vi "M--front RSw.vi"(8 "Command Info In":T1, 10 "M--front RSw":T4) -> (0 "Command Info Out":T1)   [LabVIEW 2017]
uses:
  Block Clusters/M--front RSw.ctl
  <vilib>/Rock Robotics/WPI/Framework/Command Status Info.ctl
  <vilib>/Rock Robotics/WPI/Framework/Completion Status.ctl
  <vilib>/Rock Robotics/WPI/Framework/Completion Notifier.ctl
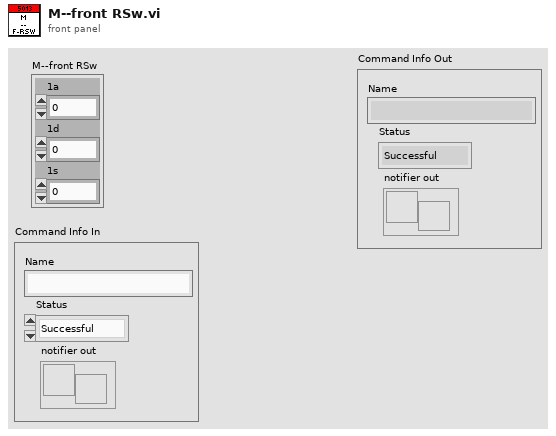
[diagram p1: front panel]
types:
  T1 = typedef "Command Status Info.ctl" = cluster{"Name":string, "Status":T2, "notifier out":T3}
  T2 = typedef "Completion Status.ctl" = enum16{"Successful", "Aborted", "Incomplete"}
  T3 = typedef "Completion Notifier.ctl" = refnum<notifier>
  T4 = typedef "M--front RSw.ctl" = cluster{"1a":dbl, "1d":dbl, "1s":dbl}
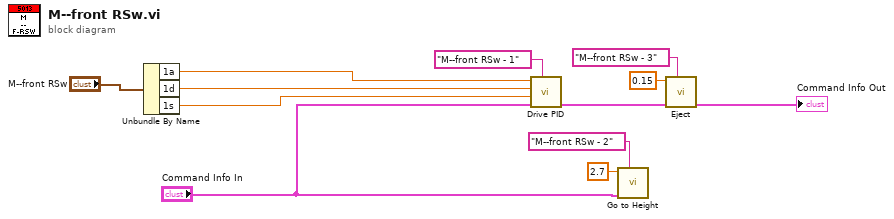
[diagram p0: block diagram]
diagram:
  n1 = Unbundle By Name("M--front RSw") -> ("1a"=w11:dbl, "1d"=w10:dbl, "1s"=w9:dbl)
  n2 = call "Drive PID.vi"("Description"="M--front RSw - 1", "Command Info In"="Command Info In", "Speed"=w9, "Distance"=w10, "Target Angle"=w11) -> ("Command Info Out"=w7:T1)  [unwired: 6 in]
  n3 = call "Go to Height.vi"("Description"="M--front RSw - 2", "Command Info In"="Command Info In", "Target Height (in)"=2.7) -> ()  [unwired: 8 in, 1 out]
  n4 = call "Eject.vi"("Description"="M--front RSw - 3", "Command Info In"=w7, "Setpoint"=0.15) -> ("Command Info Out"=→"Command Info Out":T1)  [unwired: 8 in]
